vi "STS Calculator_2014_12_09.vi"(8 "NumPts":i32=3, 9 "Hysteresis Analysis":enum32{"1st Sweep", "2nd Sweep", "Both"}(radio), 10 "Saturation Id":dbl[](array[numeric]), 11 "Vg Column":dbl[](array[numeric])) -> (0 "STS Index":dbl, 1 "NumPts 2":i32=3, 2 "XY Graph":cluster{dbl[], dbl[]}[](graph), 3 "Sub Threshold Swing":dbl, 5 "Used Points":cluster{"Vg Used":dbl[], "Id Used":dbl[]})   [LabVIEW 2015]
uses:
  <vilib>/Analysis/NI_AALPro.lvlib
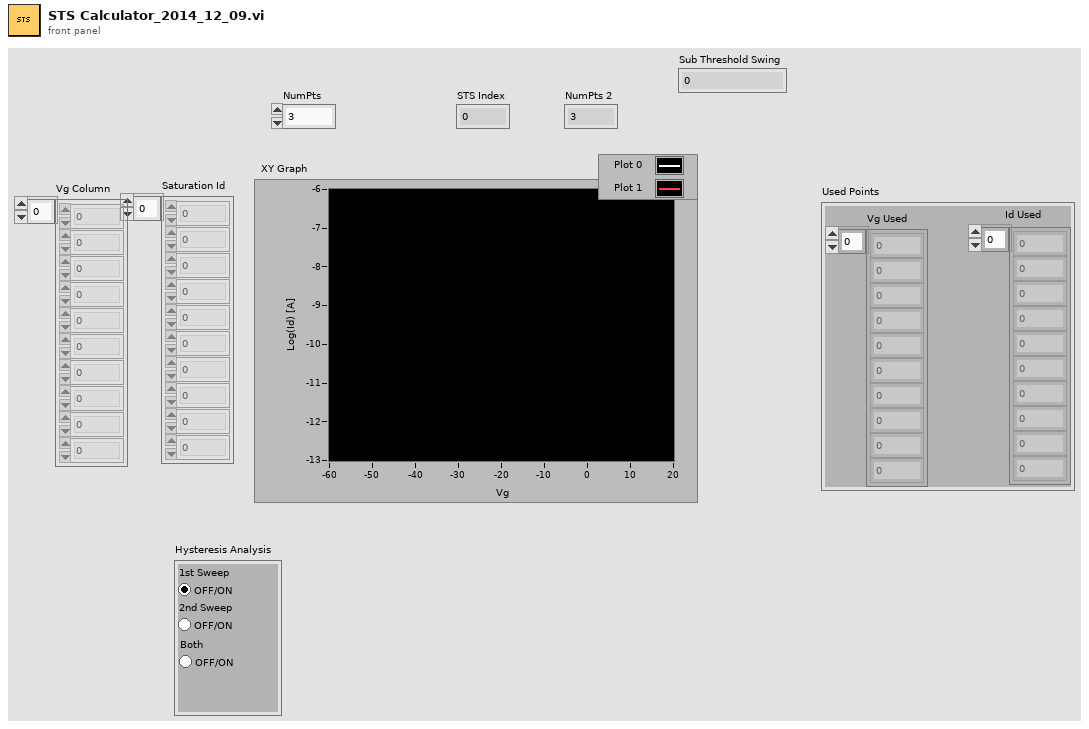
[diagram p1: front panel]
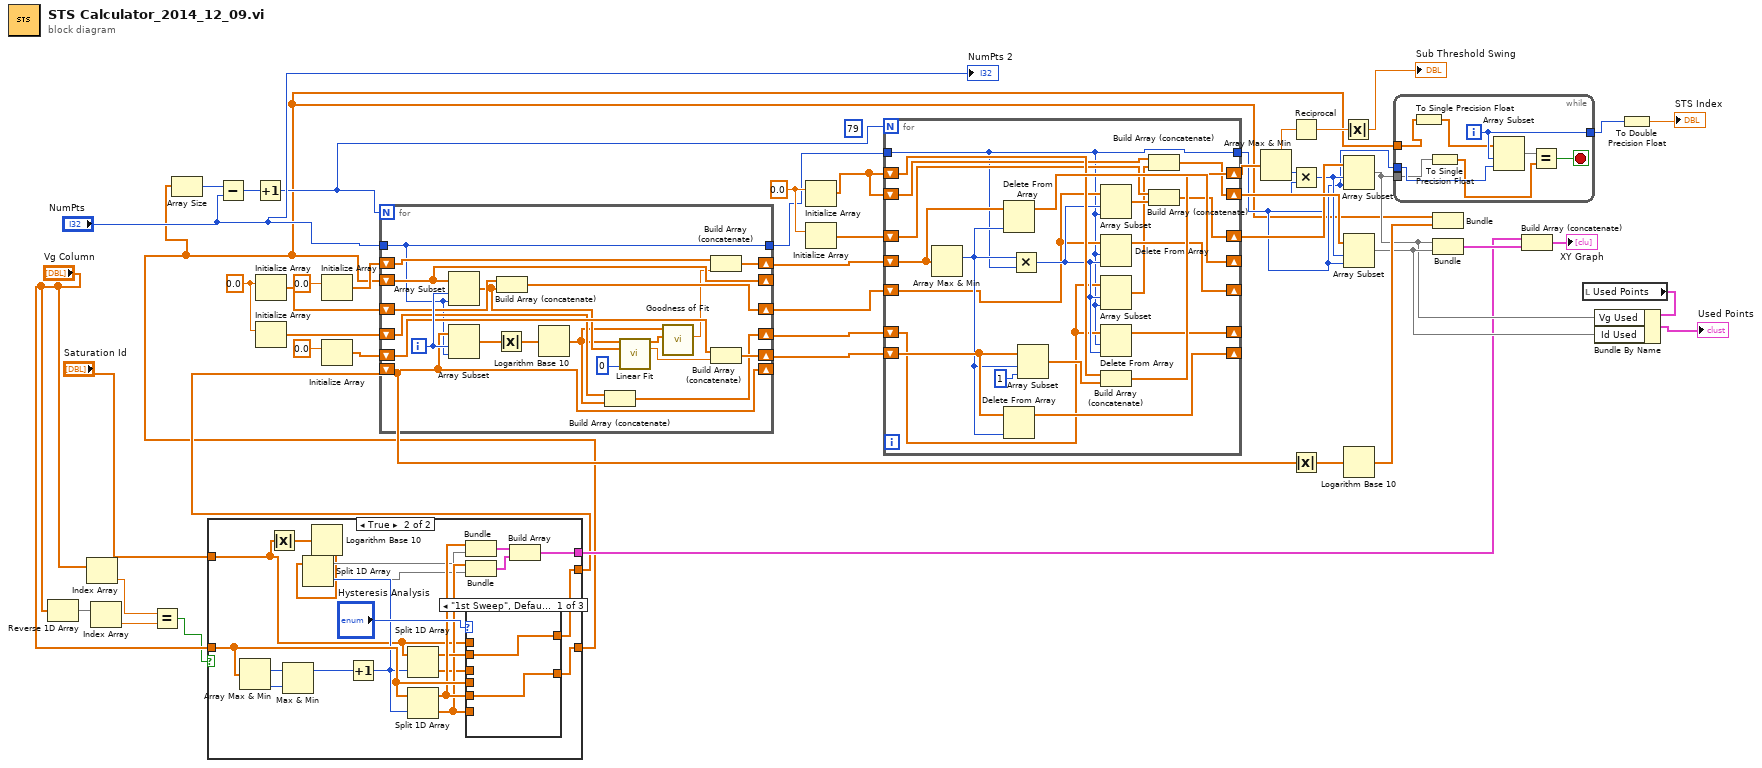
[diagram p0: block diagram]
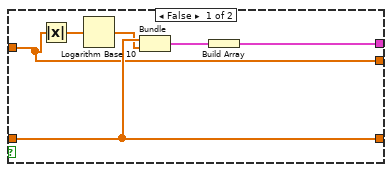
[diagram p2: hidden frame]
diagram:
  w28 = 0.0
  w34 = 0.0
  (unwired) 79
  n1 = Reverse 1D Array(array="Vg Column") -> (reversed array=w8:dbl[])
  n2 = Index Array(array="Vg Column") -> (element=w6:dbl)  [unwired: 1 in]
  n3 = Index Array(array=w8) -> (element=w7:dbl)  [unwired: 1 in]
  n4 = Equal?(x=w6, y=w7) -> (x = y?=w4:bool)
  n5 = case shown="True" w4 {
    tunnel: "Vg Column" -> [w52 w70]
    tunnel: [w52 w69] -> w1
    tunnel: "Saturation Id" -> [w49 w55]
    tunnel: [w49 w67] -> w2
    tunnel: [w51 w60] -> w3
    frame False {
      n6 = Absolute Value(x=w49) -> (abs(x)=w50:dbl[])
      n7 = Logarithm Base 10(1:w50) -> (0:w48:dbl[])
      n8 = Bundle("Vg Column"=w52, w48) -> (w53:cluster{"Vg Column":dbl[], dbl[]})  [unwired: 1 in]
      n9 = Build Array(w53) -> (w51:cluster{"Vg Column":dbl[], dbl[]}[])
    }
    frame True {
      n10 = Array Max & Min(array=w70) -> (max index (indices)=w72:i32, min index (indices)=w73:i32)  [unwired: 2 out]
      n11 = Absolute Value(x=w55) -> (abs(x)=w56:dbl[])
      n12 = Max & Min(x=w72, y=w73) -> (max(x,y)=w68:i32)  [unwired: 1 out]
      n13 = Logarithm Base 10(1:w56) -> (0:w54:dbl[])
      n14 = Increment(x=w68) -> (x+1=w59:i32)
      n15 = Split 1D Array(array=w54, index=w59) -> (first subarray=w57:dbl[], second subarray=w58:dbl[])
      n16 = Split 1D Array(array=w55, index=w59) -> (first subarray=w64:dbl[], second subarray=w62:dbl[])
      n17 = Split 1D Array(array=w70, index=w59) -> (first subarray=w65:dbl[], second subarray=w63:dbl[])
      n18 = Bundle(w65, w57) -> (w66:cluster{dbl[], dbl[]})  [unwired: 1 in]
      n19 = Bundle(w63, w58) -> (w61:cluster{dbl[], dbl[]})  [unwired: 1 in]
      n20 = case shown="\"1st Sweep\", Default" "Hysteresis Analysis" {
        tunnel: w65 -> [w74 _ _]
        tunnel: w63 -> [_ w76 _]
        tunnel: w70 -> [_ _ w79]
        tunnel: [w74 w76 w79] -> w69
        tunnel: w64 -> [w75 _ _]
        tunnel: w62 -> [_ w77 _]
        tunnel: w55 -> [_ _ w78]
        tunnel: [w75 w77 w78] -> w67
        frame "1st Sweep", Default {
        }
        frame "2nd Sweep" {
        }
        frame "Both" {
        }
      }
      n21 = Build Array(w66, w61) -> (w60:cluster{dbl[], dbl[]}[])
    }
  }
  n22 = Array Size(array=w1) -> (size(s)=w43:i32)
  n23 = Subtract(x=w43, y="NumPts") -> (x-y=w21:i32)
  n24 = Increment(x=w21) -> (x+1=w10:i32)
  n25 = Initialize Array(w34) -> (w32:dbl[])  [unwired: 1 in]
  n26 = Initialize Array(w34) -> (w33:dbl[])  [unwired: 1 in]
  n27 = Initialize Array(0.0) -> (w41:dbl[])  [unwired: 1 in]
  n28 = Initialize Array(0.0) -> (w42:dbl[])  [unwired: 1 in]
  n29 = for {
    N: w10 -> [_]
    shift-right: [w87] -> _
    shift-left: w1 -> [w87]
    shift-right: [w93] -> _
    shift-left: w2 -> [w93]
    shift-right: [w97] -> w38
    shift-left: w42 -> [w96]
    shift-right: [w95] -> w36
    shift-left: w41 -> [w94]
    tunnel: "NumPts" -> [w80]
    shift-right: [w90] -> w31
    shift-left: w33 -> [w91]
    shift-right: [w88] -> w30
    shift-left: w32 -> [w89]
    tunnel: [w80] -> w16
    i -> [w99]
    n30 = Array Subset(array=w87, index=w99, length=w80) -> (w86:dbl[])
    n31 = Array Subset(array=w93, index=w99, length=w80) -> (w81:dbl[])
    n32 = Absolute Value(x=w81) -> (abs(x)=w82:dbl[])
    n33 = Build Array (concatenate)(w89, w86) -> (w88:dbl[])
    n34 = Logarithm Base 10(1:w82) -> (0:w83:dbl[])
    n35 = Build Array (concatenate)(w91, w83) -> (w90:dbl[])
    n36 = call <vilib>:"Linear Fit.vi"("Y"=w83, "X"=w86, "method"=0) -> ("Best Linear Fit"=w85:dbl[], "slope"=w98:dbl)  [unwired: 8 in, 3 out]
    n37 = call <vilib>:"Goodness of Fit.vi"("Best Fit"=w85, "Y"=w83) -> ("R-square"=w84:dbl)  [unwired: 6 in, 3 out]
    n38 = Build Array (concatenate)(w94, w84) -> (w95:dbl[])
    n39 = Build Array (concatenate)(w96, w98) -> (w97:dbl[])
  }
  n40 = Initialize Array(w28) -> (w24:dbl[])  [unwired: 1 in]
  n41 = Initialize Array(w28) -> (w29:dbl[])  [unwired: 1 in]
  n42 = for {
    N: w10 -> [_]
    shift-right: [w119] -> _
    shift-left: w36 -> [w120]
    shift-right: [w104] -> _
    shift-left: w38 -> [w105]
    shift-right: [w116] -> w37
    shift-left: w24 -> [w115]
    shift-right: [w114] -> _
    shift-left: w31 -> [w102]
    shift-right: [w112] -> _
    shift-left: w30 -> [w101]
    tunnel: w16 -> [w100]
    shift-right: [w111] -> w27
    shift-left: w24 -> [w110]
    shift-right: [w109] -> w26
    shift-left: w29 -> [w108]
    tunnel: [w100] -> w15
    n43 = Array Max & Min(array=w120) -> (max index (indices)=w103:i32)  [unwired: 3 out]
    n44 = Delete From Array(array=w120, index=w103) -> (array with subset deleted=w119:dbl[])  [unwired: 1 in, 1 out]
    n45 = Delete From Array(array=w105, index=w103) -> (array with subset deleted=w104:dbl[])  [unwired: 1 in, 1 out]
    n46 = Multiply(x=w103, y=w100) -> (x*y=w113:i32)
    n47 = Array Subset(array=w105, index=w103, length=1) -> (w117:dbl[])
    n48 = Array Subset(array=w101, index=w113, length=w100) -> (w107:dbl[])
    n49 = Delete From Array(array=w101, length=w100, index=w113) -> (array with subset deleted=w112:dbl[])  [unwired: 1 out]
    n50 = Array Subset(array=w102, index=w113, length=w100) -> (w106:dbl[])
    n51 = Delete From Array(array=w102, length=w100, index=w113) -> (array with subset deleted=w114:dbl[])  [unwired: 1 out]
    n52 = Build Array (concatenate)(w115, w117) -> (w116:dbl[])
    n53 = Build Array (concatenate)(w110, w106) -> (w111:dbl[])
    n54 = Build Array (concatenate)(w108, w107) -> (w109:dbl[])
  }
  n55 = Array Max & Min(array=w37) -> (min value=w46:dbl, min index (indices)=w25:i32)  [unwired: 2 out]
  n56 = Reciprocal(x=w46) -> (1/x=w47:dbl)
  n57 = Multiply(x=w25, y=w15) -> (x*y=w23:i32)
  n58 = Absolute Value(x=w2) -> (abs(x)=w45:dbl[])
  n59 = Absolute Value(x=w47) -> (abs(x)=→"Sub Threshold Swing":dbl)
  n60 = Array Subset(array=w26, index=w23, length=w15) -> (w18:dbl[])
  n61 = Array Subset(array=w27, index=w23, length=w15) -> (w19:dbl[])
  n62 = Logarithm Base 10(1:w45) -> (0:w44:dbl[])
  n63 = while {
    tunnel: w1 -> [w124]
    tunnel: w18 -> [w123]
    tunnel: [w126] -> w13
    tunnel: w15 -> [w125]
    i -> [w126]
    stop <- w128 stop-if-true
    n64 = To Single Precision Float(number=w124) -> (single precision float=w122:sgl[])
    n65 = To Single Precision Float(number=w123) -> (single precision float=w121:sgl[])
    n66 = Array Subset(array=w122, index=w126, length=w125) -> (w127:sgl[])
    n67 = Equal?(x=w127, y=w121) -> (x = y?=w128:bool)
  }
  n68 = Bundle("Vg Column"=w1, w44) -> ()  [unwired: 1 in, 1 out]
  n69 = Bundle(w18, w19) -> (w22:cluster{dbl[], dbl[]})  [unwired: 1 in]
  n70 = Build Array (concatenate)(w3, w22) -> (→"XY Graph":cluster{"Vg Column":dbl[], dbl[]}[])
  n71 = local read "Used Points"() -> (w20:cluster{"Vg Used":dbl[], "Id Used":dbl[]})
  n72 = Bundle By Name(cluster=w20, "Vg Used"=w18, "Id Used"=w19) -> (→"Used Points":cluster{"Vg Used":dbl[], "Id Used":dbl[]})
  n73 = To Double Precision Float(number=w13) -> (double precision float=→"STS Index":dbl)
  "NumPts 2" <- "NumPts"
